vi "json Insert json - array path.vi"(8 "error in (no error)":errorcluster, 9 "anything":refnum<class "JSON Document.lvclass">, 10 "path":string[](array[string]), 11 "JSON Document in":refnum<class "JSON Document.lvclass">) -> (0 "error out":errorcluster, 1 "replaced?":bool, 3 "JSON Document out":refnum<class "JSON Document.lvclass">)   [LabVIEW 2015]
uses:
  JSON Document.lvclass
  json Insert - String Path.vi
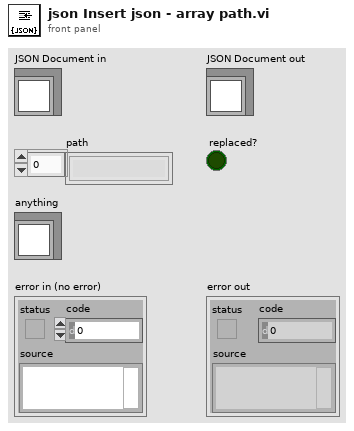
[diagram p1: front panel]
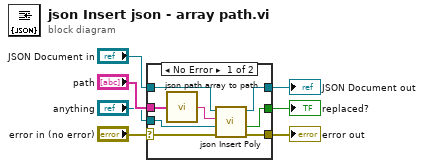
[diagram p0: block diagram]
diagram:
  n1 = case shown="No Error" "error in (no error)" {
    selector: "error in (no error)" -> [w11 w17]
    tunnel: [w12 w17] -> w3
    tunnel: [w13 w16] -> w2
    tunnel: "JSON Document in" -> [w14 w16]
    tunnel: "anything" -> [w10 _]
    tunnel: "path" -> [w9 _]
    tunnel: [w8 _] -> w1
    frame No Error {
      n2 = call "json path array to path.vi"("path"=w9) -> ("String"=w15:string)
      n3 = call-poly "json Insert Poly.vi"("error in (no error)"=w11, "anything"=w10, "path"=w15, "JSON Document in"=w14) -> ("error out"=w12:errorcluster, "replaced?"=w8:bool, "JSON Document out"=w13:refnum<class "JSON Document.lvclass">)  [unwired: 5 in]
    }
    frame Error {
    }
  }
  "error out" <- w3
  "JSON Document out" <- w2
  "replaced?" <- w1
